vi "C867_DLL_Test.vi"(8 "error in":errorcluster caption="entrée d'erreur") -> (0 "error out":errorcluster caption="sortie d'erreur")   [LabVIEW 2026]
uses:
  Controls/TypeDef_FGV.ctl
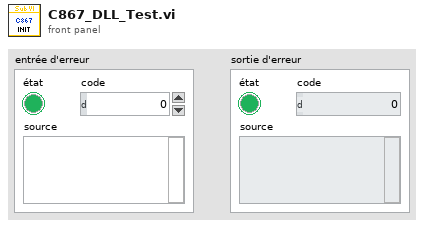
[diagram p1: front panel]
types:
  T1 = typedef "TypeDef_FGV.ctl" = enum16{"Initialize", "Write", "Read"}
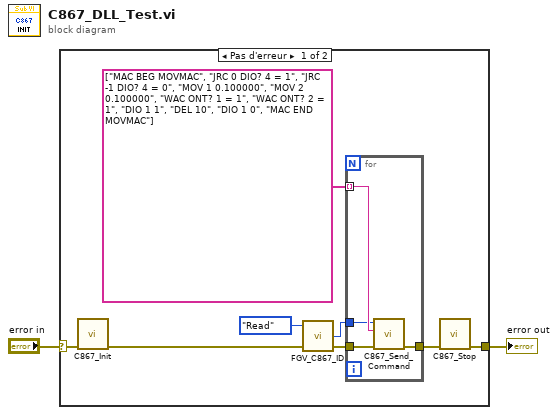
[diagram p0: block diagram]
diagram:
  n1 = case shown="Pas d'erreur" "error in" {
    selector: "error in" -> [w8 w15]
    tunnel: [w9 w15] -> w1
    frame No Error {
      n2 = call "C867_Init.vi"("error in"=w8) -> ("error out"=w4:errorcluster)  [unwired: 10 in]
      n3 = call "FGV_C867_ID.vi"("error in"=w4, "Action"=TypeDef_FGV."Read") -> ("error out"=w3:errorcluster, "ID"=w6:i32)  [unwired: 2 in]
      n4 = for {
        tunnel: string[] ["MAC BEG MOVMAC", "JRC 0 DIO? 4 = 1", "JRC -1 DIO? 4 = 0", "MOV 1 0.100000", "MOV 2 0.100000", "WAC ONT? 1 = 1", "WAC ONT? 2 = 1", "DIO 1 1", "DEL 10", "DIO 1 0", "MAC END MOVMAC"] -> [w14] mode=indexing
        tunnel: w6 -> [w13]
        tunnel: w3 -> [w12]
        tunnel: [w11] -> w7
        n5 = call "C867_Send_Command.vi"("entrée d'erreur (pas d'erreur)"=w12, "szCommand"=w14, "ID en entrée"=w13) -> ("sortie d'erreur"=w11:errorcluster)  [unwired: 6 in, 2 out]
      }
      n6 = call "C867_Stop.vi"("error in"=w7) -> ("error out"=w9:errorcluster)  [unwired: 10 in]
    }
    frame Error {
    }
  }
  "error out" <- w1
